vi "Start.vi"(0 "Arduino Connection":T1={"Baud rate (115200)"=115200, "VISA resource name"="", "Disconnect"=FALSE} {"Baud rate (115200)" min=38400 max=500000 step=1}, 1 "error in (no error)":errorcluster, 3 "Start Communication":bool) -> (2 "Arduino Conn":bool, 4 "Motor Ready":bool, 5 "Baud rate (115200)":u32, 6 "VISA resource name":refnum<visa-resource-name>, 7 "Communication":bool, 8 "error out":errorcluster, 9 "Slide":u8(slide) scale=0.0..100.0)   [LabVIEW 2018]
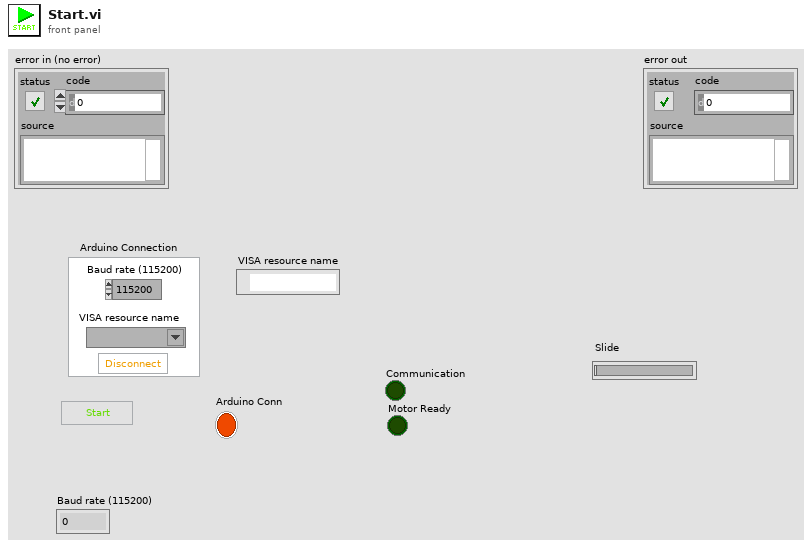
[diagram p1: front panel]
types:
  T1 = cluster{"Baud rate (115200)":u32, "VISA resource name":refnum<visa-resource-name>, "Disconnect":bool}
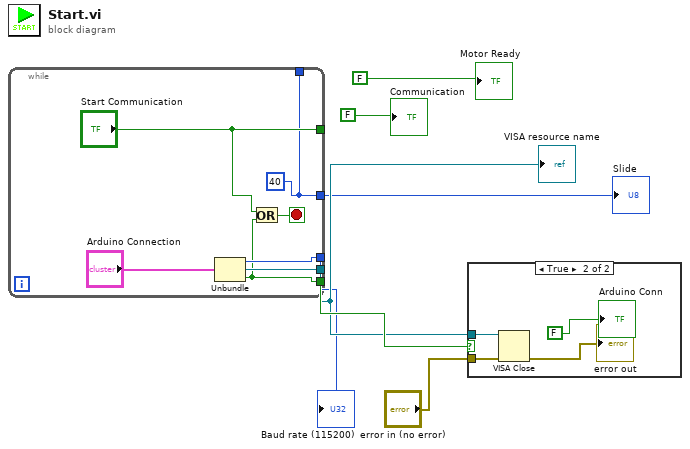
[diagram p0: block diagram]
diagram:
  n1 = while {
    tunnel: ["Start Communication"] -> _
    tunnel: [w13] -> w5
    tunnel: [w12] -> w6
    tunnel: [w10] -> w7
    tunnel: [w8] -> w2
    tunnel: [w8] -> _
    stop <- w11 stop-if-true
    w8 = u8 40 ("Slide")
    n2 = Unbundle("Arduino Connection") -> ("Baud rate (115200)"=w13:u32, "VISA resource name"=w12:refnum<visa-resource-name>, "Disconnect"=w10:bool)
    n3 = Or(x="Start Communication", y=w10) -> (x .or. y?=w11:bool)
  }
  "Baud rate (115200)" <- w5
  "VISA resource name" <- w6
  "Slide" <- w2
  n4 = case shown="True" w7 {
    tunnel: w6 -> [_ w18]
    tunnel: "error in (no error)" -> [_ w16]
    frame False {
    }
    frame True {
      n5 = VISA Close(VISA resource name=w18, error in (no error)=w16) -> (error out=→"error out":errorcluster)
      "Arduino Conn" <- FALSE ("Arduino Conn")
    }
  }
  "Communication" <- FALSE ("Communication")
  "Motor Ready" <- FALSE ("Motor Ready")
